vi "getState.vi"(8 "error in (no error)":errorcluster, 11 "ReadySate in":refnum<class "ReadySate.lvclass">) -> (0 "error out":errorcluster, 2 "DeviceStatus":T1, 3 "ReadySate out":refnum<class "ReadySate.lvclass">)   [LabVIEW 2016, in "ReadySate.lvclass"]
uses:
  ReadySate.lvclass
  Typedefs/DeviceStatus.ctl
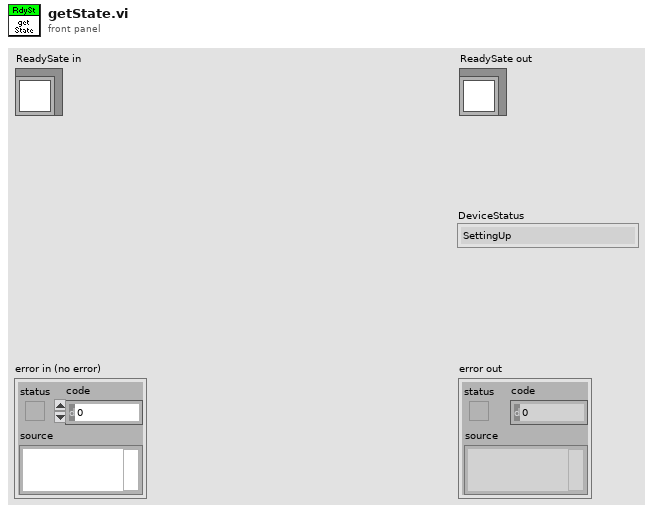
[diagram p1: front panel]
types:
  T1 = typedef "DeviceStatus.ctl" = enum16{"SettingUp", "Ready", "Offline", "Fault"}
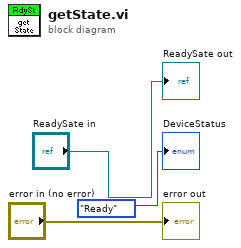
[diagram p0: block diagram]
diagram:
  "error out" <- "error in (no error)"
  "ReadySate out" <- "ReadySate in"
  "DeviceStatus" <- DeviceStatus."Ready" ("DeviceStatus")
